vi "Unix epoch time to timestamp.vi"(10 "Precision":T1=enum."Milliseconds", 11 "Unix epoch time":u64) -> (2 "Time Stamp (UTC)":timestamp format="%<%H:%M:%S%3u\n%Y/%m/%d>T", 3 "Time Stamp":timestamp format="%<%H:%M:%S%3u\n%Y/%m/%d>T")   [LabVIEW 2018, in "InfluxDB Client.lvlib"]
doc: "Convert Unix epoch time to the LabVIEW timestamp format."
uses:
  Controls/Precision.ctl
  InfluxDB Client.lvlib
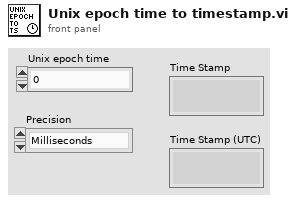
[diagram p1: front panel]
types:
  T1 = typedef "InfluxDB Client.lvlib/Precision.ctl" = enum16{"Seconds", "Milliseconds", "Nanoseconds"}
  T2 = typedef "LVDateTimeRec.ctl" = cluster{"fractional second":dbl, "second":i32, "minute":i32, "hour":i32, "day of month":i32, "month":i32, "year":i32, "day of week":i32, "day of year":i32, "DST":i32}
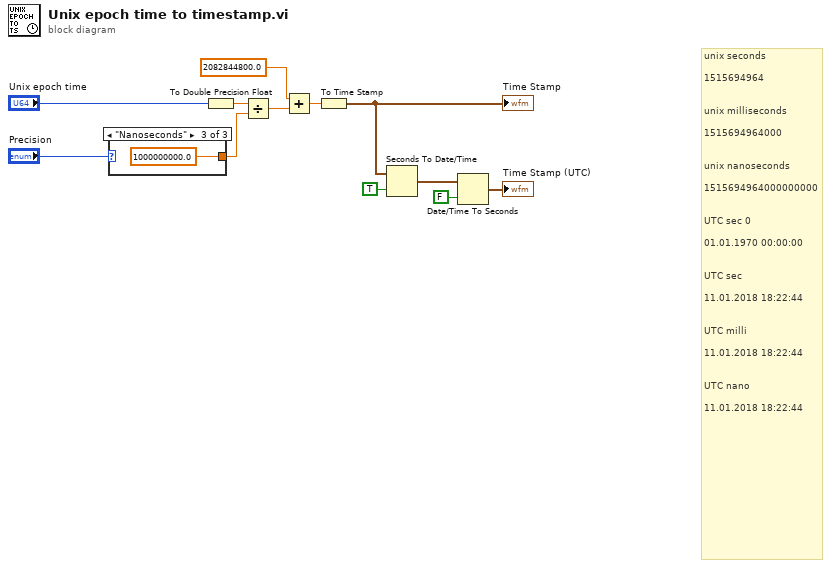
[diagram p0: block diagram]
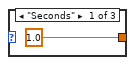
[diagram p2: hidden frame]
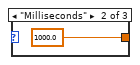
[diagram p3: hidden frame]
diagram:
  # "unix seconds\n\n1515694964 \n\n\nunix milliseconds\n\n1515694964000 \n\n\nunix nanoseconds\n\n1515694964000000000 \n\n\nUTC sec 0\n\n01.01.1970 00:00:00 \n\n\nUTC sec\n\n11.01.2018 18:22:44 \n\n\nUTC milli\n\n11.01.2018 18:22:44 \n\n\nUTC nano\n\n11.01.2018 18:22:44"
  n1 = case shown="\"Nanoseconds\"" "Precision" {
    tunnel: [1.0 ("Database name") 1000.0 ("Database name") 1000000000.0 ("Database name")] -> w9
    frame "Seconds" {
    }
    frame "Milliseconds" {
    }
    frame "Nanoseconds" {
    }
  }
  n2 = To Double Precision Float(number="Unix epoch time") -> (double precision float=w10:dbl)
  n3 = Divide(x=w10, y=w9) -> (x/y=w8:dbl)
  n4 = Add(x=2082844800.0, y=w8) -> (x+y=w7:dbl)
  n5 = To Time Stamp(1:w7) -> (0:w3:timestamp)
  "Time Stamp" <- w3
  n6 = Seconds To Date/Time(time stamp (now)=w3, to UTC (F)=TRUE) -> (date time rec=w5:T2)
  n7 = Date/Time To Seconds(1:FALSE ("is UTC (F)"), 2:w5) -> (0:→"Time Stamp (UTC)":timestamp)
